vi "Part 1.vi"(11 "Input":string) -> (3 "Output":i64)   [LabVIEW 2021]
uses:
  <userlib>/_OpenG.lib/string/string.llb/Convert EOLs (String)__ogtk.vi
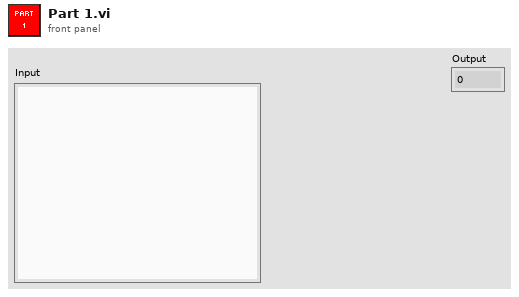
[diagram p1: front panel]
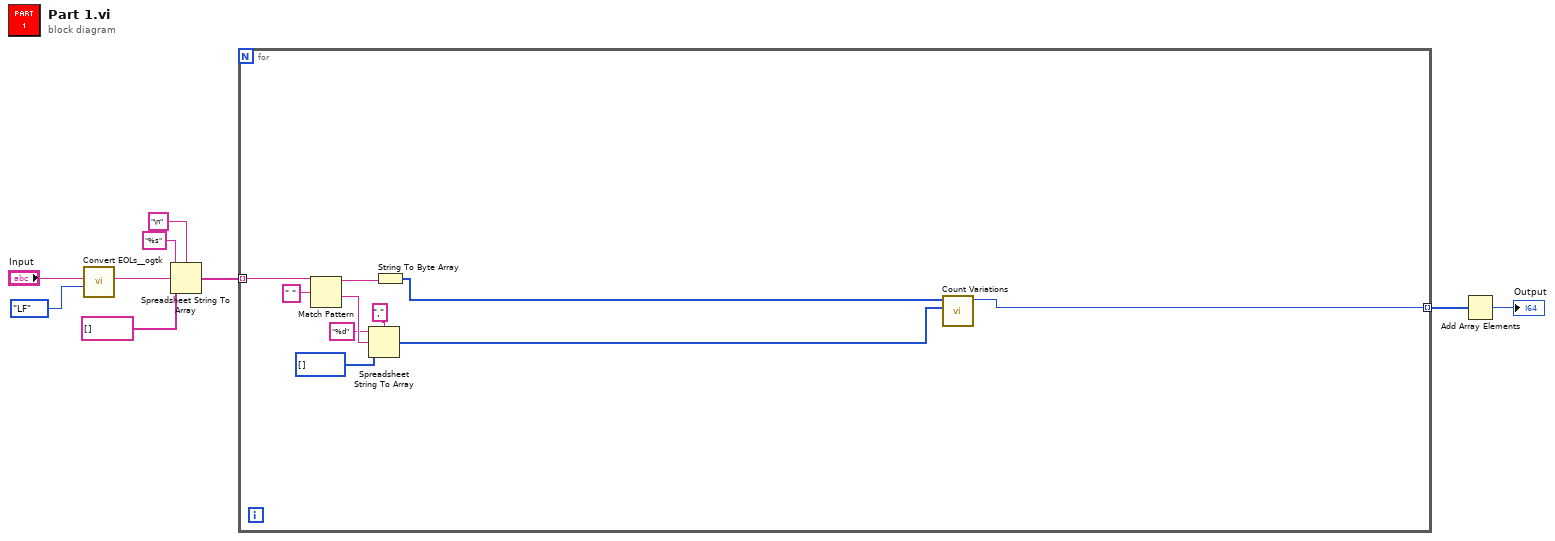
[diagram p0: block diagram]
diagram:
  n1 = call-poly <userlib>:"Convert EOLs__ogtk.vi"("Convert to:"=enum16{"CR", "LF", "CRLF"}."LF", "String in"="Input") -> ("String out"=w5:string)  [unwired: 9 in]
  n2 = Spreadsheet String To Array(delimiter (Tab)="\n", format string="%s", spreadsheet string=w5, array type (2D Dbl)=string[] []) -> (array=w3:string[])
  n3 = for {
    tunnel: w3 -> [w19] mode=indexing
    tunnel: [w13] -> w2 mode=indexing
    n4 = Match Pattern(string=w19, regular expression=" ") -> (before substring=w11:string, after substring=w17:string)  [unwired: 1 in, 2 out]
    n5 = Spreadsheet String To Array(delimiter (Tab)=",", format string="%d", spreadsheet string=w17, array type (2D Dbl)=i64[] []) -> (array=w14:i64[])
    n6 = String To Byte Array(string=w11) -> (unsigned byte array=w10:u8[])
    n7 = call "Count Variations.vi"("Array"=w14, "unsigned byte array"=w10) -> ("Numeric"=w13:i64)  [unwired: 9 in]
  }
  n8 = Add Array Elements(numeric array=w2) -> (sum=→"Output":i64)
